vi "GenerateGeneric.vi"(9 "PolyVI Refnum":refnum<vi>, 11 "actual vi":refnum<vi>) -> (3 "error out":errorcluster)   [LabVIEW 2013]
uses:
  <vilib>/NI/Tag Bus/tag/Data Type.ctl
  generic_type_definition.ctl
  <vilib>/Utility/VariantDataType/Type.ctl
  <vilib>/Utility/traverseref.llb/TRef TravTarget.ctl
  <vilib>/Utility/traverseref.llb/VI Scripting - Traverse.lvlib
  <vilib>/NI/Tag Bus/tag/tag descriptor.lvclass
  <vilib>/Utility/VariantDataType/VariantType.lvlib
panel:
  in  "multiple values":bool
  in  "Data Type":T1
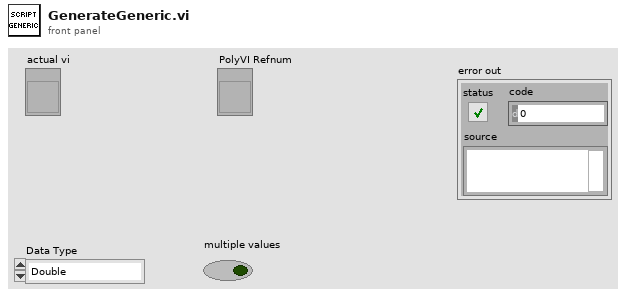
[diagram p1: front panel]
types:
  T1 = typedef "tag bus.lvlib/tag descriptor.lvclass/Data Type.ctl" = enum16{"Double", "Single", "I64", "I32", "I16", "I8", "U64", "U32", "U16", "U8", "Boolean", "String", "Array of Double", "Array of Single", "Array of I64", "Array of I32", "Array of I16", "Array of I8", "Array of U64", "Array of U32", "Array of U16", "Array of U8", "Array of Boolean", "Array of String"}
  T2 = typedef "VariantType.lvlib/Type.ctl" = enum8{"Invalid Type", "Void", "I8", "I16", "I32", "I64", "U8", "U16", "U32", "U64", "Single Float", "Double Float", "Extended Float", "Single Complex", "Double Complex", "Extended Complex", "Enum U8", "Enum U16", "Enum U32", "Enum U64", "Single Float With Unit", "Double Float With Unit", "Extended Float With Unit", "Single Complex with Unit", "Double Complex with Unit", "Extended Complex with Unit", "Boolean", "String", "Path", "Picture", "Tag", "Array", "Cluster", "Variant", "LV Variant", "Waveform", "Timestamp", "Digital Waveform", "Digital Data", "ExpressData", "Refnum", "External Data", "VI", "Poly VI", "LabVIEW Class Instance", "Fixed Point"}
  T3 = typedef "TRef TravTarget.ctl" = enum16{"FP", "BD", "Other"}
  T4 = typedef "generic_type_definition.ctl" = cluster{"name":string, "Type Enum":T2, "path (cluster)":path, "element type (array)":T2, "cluster of arrays":bool, "array of cluster of arrays":bool}
  T5 = cluster{"VIPath":path, "Menu Name":string, "Selector Name":string}[]
  T6 = cluster{"VIPath":path, "Menu Name":string, "Selector Name":string}
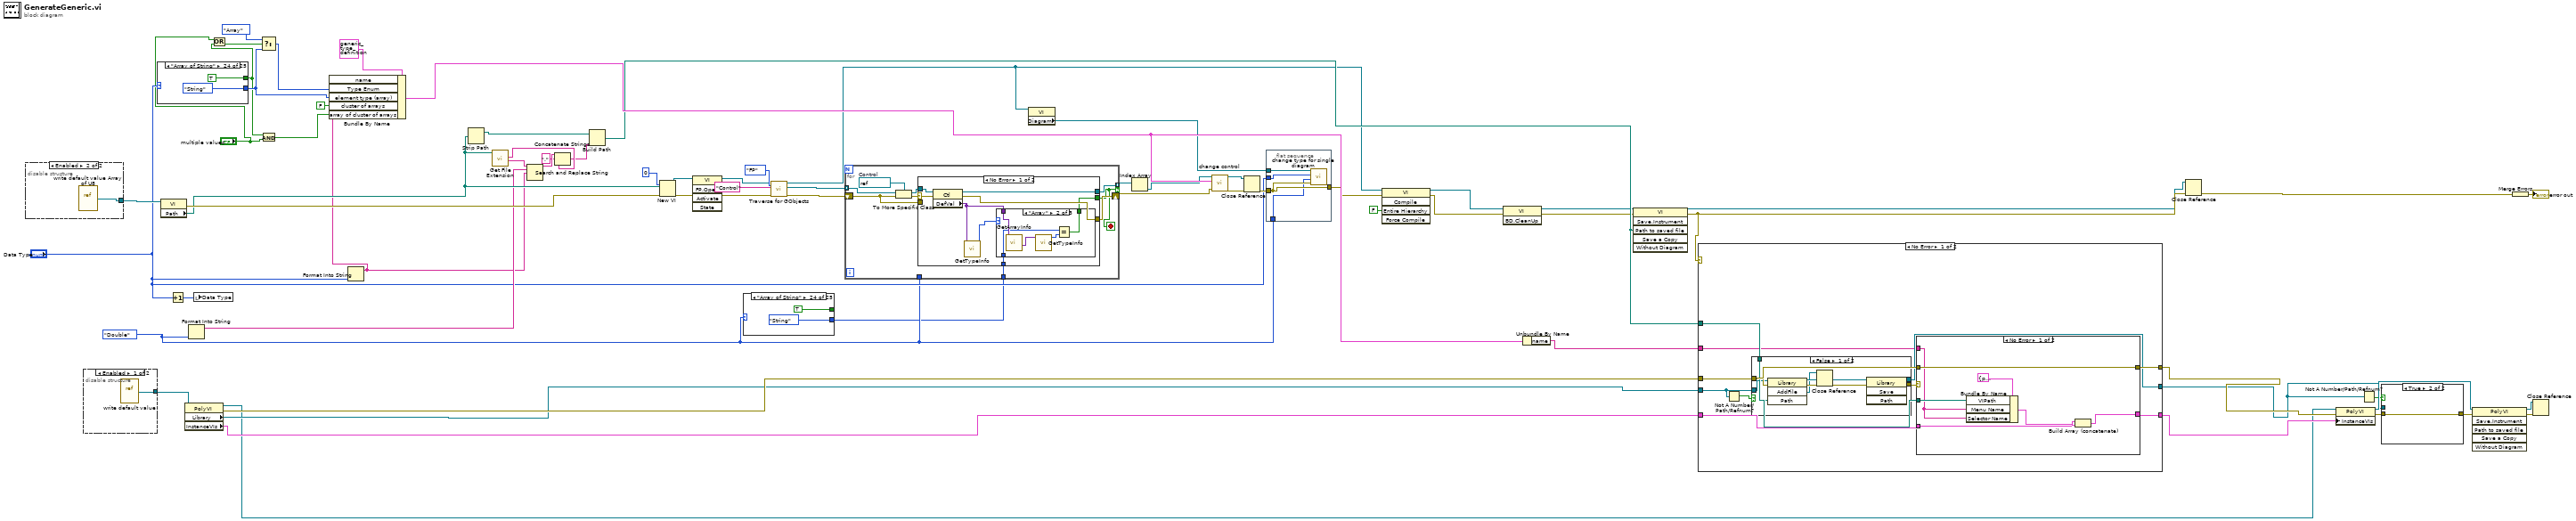
[diagram p0: block diagram]
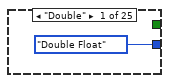
[diagram p2: hidden frame]
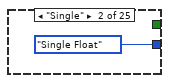
[diagram p3: hidden frame]
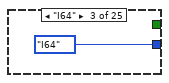
[diagram p4: hidden frame]
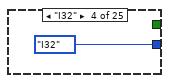
[diagram p5: hidden frame]
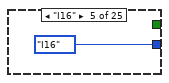
[diagram p6: hidden frame]
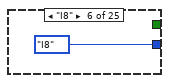
[diagram p7: hidden frame]
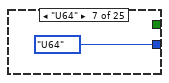
[diagram p8: hidden frame]
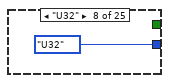
[diagram p9: hidden frame]
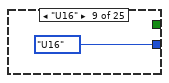
[diagram p10: hidden frame]
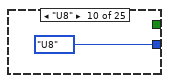
[diagram p11: hidden frame]
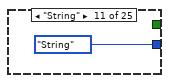
[diagram p12: hidden frame]
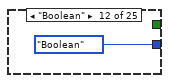
[diagram p13: hidden frame]
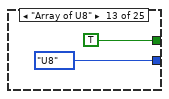
[diagram p14: hidden frame]
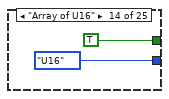
[diagram p15: hidden frame]
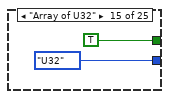
[diagram p16: hidden frame]
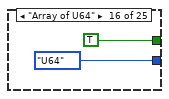
[diagram p17: hidden frame]
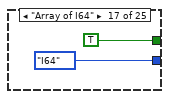
[diagram p18: hidden frame]
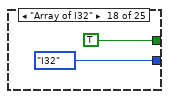
[diagram p19: hidden frame]
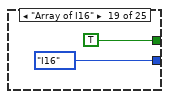
[diagram p20: hidden frame]
diagram:
  w5 = Data_Type."Double" ("element")
  n1 = disable-structure shown="Enabled" {
    disable-tunnel: ["actual vi" w69] -> w49
    frame Disabled {
    }
    frame Enabled {
      n2 = vi-ref <vilib>:"write default value Array of U8.vi"() -> (w69:refnum<vi>)
    }
  }
  n3 = disable-structure shown="Enabled" {
    disable-tunnel: [w70 "PolyVI Refnum"] -> w65
    frame Enabled {
      n4 = vi-ref <vilib>:"write default value.vi"() -> (w70:refnum<vi>)
    }
    frame Disabled {
    }
  }
  n5 = case shown="\"Array of String\"" "Data Type" {
    tunnel: [Type."Double Float" ("Type Enum") Type."Single Float" ("Type Enum") Type."I64" ("Type Enum") Type."I32" ("Type Enum") Type."I16" ("Type Enum") Type."I8" ("Type Enum") Type."U64" ("Type Enum") Type."U32" ("Type Enum") Type."U16" ("Type Enum") Type."U8" ("Type Enum") Type."String" ("Type Enum") Type."Boolean" ("Type Enum") Type."U8" ("Type Enum") Type."U16" ("Type Enum") Type."U32" ("Type Enum") Type."U64" ("Type Enum") Type."I64" ("Type Enum") Type."I32" ("Type Enum") Type."I16" ("Type Enum") Type."I8" ("Type Enum") Type."Double Float" ("Type Enum") Type."Single Float" ("Type Enum") Type."Boolean" ("Type Enum") Type."String" ("Type Enum") Type."Invalid Type" ("Type Enum")] -> w14
    tunnel: [_ _ _ _ _ _ _ _ _ _ _ _ TRUE TRUE TRUE TRUE TRUE TRUE TRUE TRUE TRUE TRUE TRUE TRUE _] -> w9
    frame "Double" {
    }
    frame "Single" {
    }
    frame "I64" {
    }
    frame "I32" {
    }
    frame "I16" {
    }
    frame "I8" {
    }
    frame "U64" {
    }
    frame "U32" {
    }
    frame "U16" {
    }
    frame "U8" {
    }
    frame "String" {
    }
    frame "Boolean" {
    }
    frame "Array of U8" {
    }
    frame "Array of U16" {
    }
    frame "Array of U32" {
    }
    frame "Array of U64" {
    }
    frame "Array of I64" {
    }
    frame "Array of I32" {
    }
    frame "Array of I16" {
    }
    frame "Array of I8" {
    }
    frame "Array of Double" {
    }
    frame "Array of Single" {
    }
    frame "Array of Boolean" {
    }
    frame "Array of String" {
    }
    frame Default {
    }
  }
  n6 = property class="VI"(reference=w49) -> (error out=w67:errorcluster, "Path"=w66:path)  [unwired: 1 in, 1 out]
  n7 = Increment(x="Data Type") -> (x+1=w15:T1)
  n8 = property class="PolyVI"(reference=w65) -> (reference out=w52:refnum<vi>, error out=w63:errorcluster, "Library"=w61:refnum<vi>, "InstanceVIs"=w56:T5)  [unwired: 1 in]
  n9 = Format Into String(w5) -> (resulting string=w48:string)  [unwired: 3 in, 1 out]
  n10 = local write "Data Type"(w15) -> ()
  n11 = Or(x="multiple values", y=w9) -> (x .or. y?=w11:bool)
  n12 = Select(t=Type."Array", s=w11, f=w14) -> (s? t:f=w12:T2)
  n13 = And(x=w9, y="multiple values") -> (x .and. y?=w8:bool)
  n14 = Format Into String("Data Type") -> (resulting string=w45:string)  [unwired: 3 in, 1 out]
  n15 = Bundle By Name(cluster=T4 {"name"="", "Type Enum"=enum."Invalid Type", "path (cluster)"=path "", "element type (array)"=enum."Invalid Type", "cluster of arrays"=FALSE, "array of cluster of arrays"=FALSE}, "name"=w45, "Type Enum"=w12, "element type (array)"=w14, "cluster of arrays"=FALSE, "array of cluster of arrays"=w8) -> (w46:T4)
  n16 = Strip Path(path=w66) -> (stripped path=w26:path)  [unwired: 1 out]
  n17 = call <vilib>:"Get File Extension.vi"("file"=w66) -> ("filename without extension"=w31:string, "lowercase file extension"=w28:string)  [unwired: 7 in, 2 out]
  n18 = Search and Replace String(input string=w31, search string=w48, replace string=w45) -> (result string=w30:string)  [unwired: 5 in, 3 out]
  n19 = Concatenate Strings(w30, "." ("string"), w28) -> (w27:string)
  n20 = Build Path(base path=w26, name or relative path=w27) -> (appended path=w32:path)
  n21 = New VI(7:u32 0 ("options"), 8:w67, 10:w66) -> (0:w39:errorcluster, 3:w40:refnum<vi>)  [unwired: 4 in]
  n22 = invoke class="VI" method="FP.Open"(reference=w40) -> (reference out=w21:refnum<vi>)  [unwired: 4 in, 4 out]
  n23 = case shown="\"Array of String\"" w5 {
    tunnel: [Type."Double Float" ("Type Enum") Type."Single Float" ("Type Enum") Type."I64" ("Type Enum") Type."I32" ("Type Enum") Type."I16" ("Type Enum") Type."I8" ("Type Enum") Type."U64" ("Type Enum") Type."U32" ("Type Enum") Type."U16" ("Type Enum") Type."U8" ("Type Enum") Type."String" ("Type Enum") Type."Boolean" ("Type Enum") Type."U8" ("Type Enum") Type."U16" ("Type Enum") Type."U32" ("Type Enum") Type."U64" ("Type Enum") Type."I64" ("Type Enum") Type."I32" ("Type Enum") Type."I16" ("Type Enum") Type."I8" ("Type Enum") Type."Double Float" ("Type Enum") Type."Single Float" ("Type Enum") Type."Boolean" ("Type Enum") Type."String" ("Type Enum") Type."Invalid Type" ("Type Enum")] -> w4
    tunnel: [_ _ _ _ _ _ _ _ _ _ _ _ TRUE TRUE TRUE TRUE TRUE TRUE TRUE TRUE TRUE TRUE TRUE TRUE _] -> _
    frame "Double" {
    }
    frame "Single" {
    }
    frame "I64" {
    }
    frame "I32" {
    }
    frame "I16" {
    }
    frame "I8" {
    }
    frame "U64" {
    }
    frame "U32" {
    }
    frame "U16" {
    }
    frame "U8" {
    }
    frame "String" {
    }
    frame "Boolean" {
    }
    frame "Array of U8" {
    }
    frame "Array of U16" {
    }
    frame "Array of U32" {
    }
    frame "Array of U64" {
    }
    frame "Array of I64" {
    }
    frame "Array of I32" {
    }
    frame "Array of I16" {
    }
    frame "Array of I8" {
    }
    frame "Array of Double" {
    }
    frame "Array of Single" {
    }
    frame "Array of Boolean" {
    }
    frame "Array of String" {
    }
    frame Default {
    }
  }
  n24 = call <vilib>:"Traverse for GObjects.vi"("Traverse Target"=TRef_TravTarget."FP", "error in (no error)"=w39, "Class Name"="Control", "VI Refnum"=w21) -> ("error out"=w43:errorcluster, "References"=w42:refnum<vi>[], "dup VI Refnum"=w17:refnum<vi>)  [unwired: 4 in, 1 out]
  n25 = for {
    tunnel: w42 -> [w154] mode=indexing
    tunnel: [w150] -> w23 mode=indexing if=w147
    shift-right: [w149] -> w20
    shift-left: w43 -> [w148]
    tunnel: w5 -> [_]
    tunnel: w4 -> [w146]
    stop <- w147 stop-if-true
    w153 = refnum<vi> refnum  # Control
    n26 = To More Specific Class(target class=w153, reference=w154, error in=w148) -> (specific class reference=w151:refnum<vi>, error out=w152:errorcluster)
    n27 = case shown="No Error" w152 {
      selector: w152 -> [w161 _]
      tunnel: w151 -> [w162 _]
      tunnel: [w157 FALSE] -> w147
      tunnel: [w160 _] -> w150
      tunnel: [w159 w170] -> w149
      tunnel: w148 -> [_ w170]
      tunnel: w146 -> [w155 _]
      frame No Error {
        n28 = property class="Ctl"(reference=w162, error in=w161) -> (reference out=w160:refnum<vi>, error out=w159:errorcluster, "DefVal"=w156:variant)
        n29 = call <vilib>:"GetTypeInfo.vi"("Variant"=w156) -> ("Type Enum"=w158:T2)  [unwired: 6 in, 4 out]
        n30 = case shown="\"Array\"" w158 {
          tunnel: [FALSE w165 TRUE] -> w157
          tunnel: w156 -> [_ w168 _]
          tunnel: w155 -> [_ w164 _]
          frame Default {
          }
          frame "Array" {
            n31 = call <vilib>:"GetArrayInfo.vi"("Variant"=w168) -> ("ArrayElement"=w167:variant)  [unwired: 7 in, 3 out]
            n32 = call <vilib>:"GetTypeInfo.vi"("Variant"=w167) -> ("Type Enum"=w166:T2)  [unwired: 6 in, 4 out]
            n33 = Equal?(x=w164, y=w166) -> (x = y?=w165:bool)
          }
          frame "Double Float" {
          }
        }
      }
      frame Error {
        # "death of a parent"
      }
    }
  }
  n34 = property class="VI"(reference=w17) -> ("Diagram"=w16:refnum<vi>)  [unwired: 1 in, 2 out]
  n35 = Index Array(array=w23) -> (element=w22:refnum<vi>)  [unwired: 1 in]
  n36 = call "change control.vi"("error in (no error)"=w20, "type definition"=w46, "Control in"=w22) -> ("error out"=w25:errorcluster, "control out"=w24:refnum<vi>)  [unwired: 7 in]
  n37 = Close Reference(reference=w24, error in (no error)=w25) -> (error out=w19:errorcluster)
  n38 = flat-sequence {
    tunnel: w19 -> [w175]
    tunnel: [w175] -> w18
    tunnel: w16 -> [w174]
    tunnel: "Data Type" -> [w173]
    tunnel: w5 -> [w172]
    frame #0 {
      n39 = call "change type for single diagram.vi"("error in (no error)"=w175, "old type"=w172, "new type"=w173, "Diagram in"=w174) -> ()  [unwired: 8 in]
    }
  }
  n40 = invoke class="VI" method="Compile"(reference=w17, error in=w18, "Entire Hierarchy"=FALSE ("Compile Entire Hierarchy (F)")) -> (reference out=w2:refnum<vi>, error out=w36:errorcluster)  [unwired: 2 in, 3 out]
  n41 = invoke class="VI" method="BD.CleanUp"(reference=w2, error in=w36) -> (reference out=w1:refnum<vi>, error out=w3:errorcluster)  [unwired: 1 in, 1 out]
  n42 = Unbundle By Name(w46) -> ("name"=w33:string)
  n43 = invoke class="VI" method="Save.Instrument"(reference=w1, error in=w3, "Path to saved file"=w32) -> (reference out=w34:refnum<vi>, error out=w35:errorcluster)  [unwired: 3 in, 4 out]
  n44 = case shown="No Error" w35 {
    tunnel: [w184 w208] -> w58
    tunnel: w63 -> [w183 w208]
    tunnel: w61 -> [w177 w207]
    tunnel: [w180 w207] -> w51
    tunnel: [w181 w206] -> w53
    tunnel: w56 -> [w182 w206]
    tunnel: w32 -> [w179 _]
    tunnel: w33 -> [w178 _]
    frame No Error {
      n45 = Not A Number/Path/Refnum?(number/path/refnum=w177) -> (NaN/Path/Refnum?=w176:bool)
      n46 = case shown="False" w176 {
        tunnel: [w190 w196] -> w185
        tunnel: w183 -> [w189 w196]
        tunnel: [w188 w195] -> w180
        tunnel: w179 -> [w187 _]
        tunnel: w177 -> [w186 w195]
        frame False {
          n47 = invoke class="Library" method="AddFile"(reference=w186, error in=w189, "Path"=w187) -> (reference out=w193:refnum<vi>, error out=w194:errorcluster, "AddFile"=w191:refnum<vi>)  [unwired: 1 in, 1 out]
          n48 = Close Reference(reference=w191, error in (no error)=w194) -> (error out=w192:errorcluster)
          n49 = invoke class="Library" method="Save"(reference=w193, error in=w192) -> (reference out=w188:refnum<vi>, error out=w190:errorcluster)  [unwired: 2 in, 2 out]
        }
        frame True {
        }
      }
      n50 = case shown="No Error" w185 {
        tunnel: [w203 w205] -> w184
        tunnel: w183 -> [w203 w205]
        tunnel: w182 -> [w199 w204]
        tunnel: [w201 w204] -> w181
        tunnel: w179 -> [w198 _]
        tunnel: w178 -> [w197 _]
        frame No Error {
          n51 = Bundle By Name(cluster=T6 {"VIPath"=path "", "Menu Name"="", "Selector Name"=""}, "VIPath"=w198, "Menu Name"=w197, "Selector Name"=w197) -> (w200:T6)
          n52 = Build Array (concatenate)(w199, w200) -> (w201:T5)
        }
        frame Error {
        }
      }
    }
    frame Error {
    }
  }
  n53 = Close Reference(reference=w34, error in (no error)=w35) -> (error out=w64:errorcluster)
  n54 = property class="PolyVI"(reference=w52, error in=w58, "InstanceVIs"=w53) -> (reference out=w54:refnum<vi>, error out=w55:errorcluster)
  n55 = Not A Number/Path/Refnum?(number/path/refnum=w51) -> (NaN/Path/Refnum?=w50:bool)
  n56 = case shown="True" w50 {
    tunnel: [w212 w214] -> w57
    tunnel: w55 -> [w210 w214]
    tunnel: w51 -> [w209 _]
    frame False {
      n57 = invoke class="Library" method="Save"(reference=w209, error in=w210) -> (reference out=w211:refnum<vi>, error out=w213:errorcluster)  [unwired: 2 in, 2 out]
      n58 = Close Reference(reference=w211, error in (no error)=w213) -> (error out=w212:errorcluster)
    }
    frame True {
    }
  }
  n59 = invoke class="PolyVI" method="Save.Instrument"(reference=w54, error in=w57) -> (reference out=w59:refnum<vi>, error out=w60:errorcluster)  [unwired: 4 in, 4 out]
  n60 = Merge Errors(w64) -> (→"error out":errorcluster)
  n61 = Close Reference(reference=w59, error in (no error)=w60) -> ()  [unwired: 1 out]
